vi "MotorPasso_140319.vi"() -> ()   [LabVIEW 2016]
panel:
  in  "MOTOR 1":bool=TRUE
  in  "?":bool
  in  "Posição Final (Graus)":dbl
  in  "Posição Inicial (Graus)":dbl
  # "SENTIDO"
  # "Esquerda"
  # "Direita"
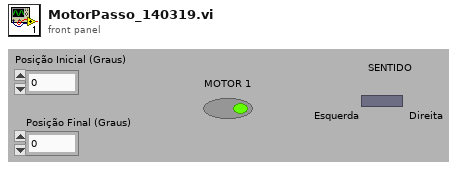
[diagram p1: front panel]
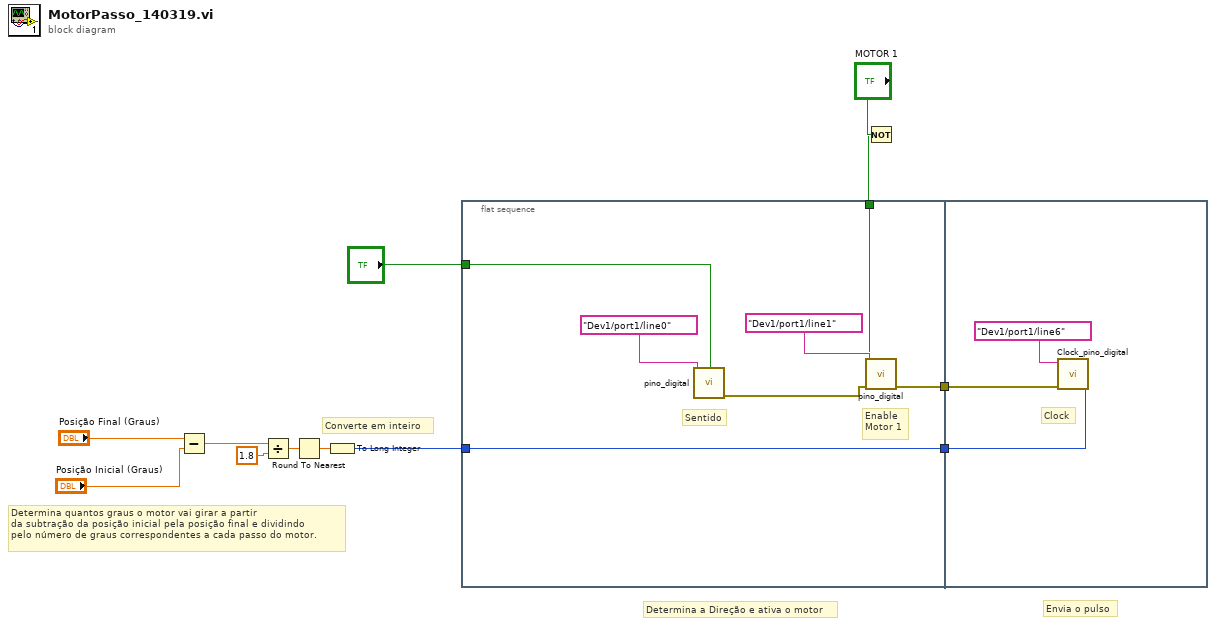
[diagram p0: block diagram]
diagram:
  # "Envia o pulso"
  # "Determina a Direção e ativa o motor"
  # "Converte em inteiro"
  # "Determina quantos graus o motor vai girar a partir\nda subtração da posição inicial pela posição final e dividindo \npelo número de graus correspondentes a cada passo do motor."
  n1 = Subtract(x="Posição Final (Graus)", y="Posição Inicial (Graus)") -> (x-y=w10:dbl)
  n2 = Divide(x=w10, y=1.8) -> (x/y=w11:dbl)
  n3 = Round To Nearest(number=w11) -> (nearest integer value=w7:dbl)
  n4 = To Long Integer(number=w7) -> (32bit integer=w4:i32)
  n5 = flat-sequence {
    tunnel: "?" -> [w18]
    tunnel: w1 -> [w16]
    tunnel: [w15] -> w5
    tunnel: w4 -> [w15]
    tunnel: [w13] -> w3
    tunnel: w5 -> [w22]
    tunnel: w3 -> [w20]
    frame #0 {
      # "Enable\nMotor 1"
      # "Sentido"
      n6 = call "pino_digital.vi"("data"=w18, "lines"=tag "Dev1/port1/line0") -> ("error out"=w14:errorcluster)  [unwired: 9 in]
      n7 = call "pino_digital.vi"("error in"=w14, "data"=w16, "lines"=tag "Dev1/port1/line1") -> ("error out"=w13:errorcluster)  [unwired: 8 in]
    }
    frame #1 {
      # "Clock"
      n8 = call "Clock_pino_digital.vi"("N loops"=w22, "error in"=w20, "lines"=tag "Dev1/port1/line6") -> ()  [unwired: 8 in, 1 out]
    }
  }
  n9 = Not(x="MOTOR 1") -> (.not. x?=w1:bool)
